vi "Binary Number Mantissa and Exponent (U64).vi"(7 "Binary Number":u64 format="%064b", 9 "Input Valid":bool=TRUE) -> (6 "Exponent (-N)":u8, 8 "Mantissa (M)":u64 format="%.0b", 10 "Output Valid":bool=TRUE)   [LabVIEW 2011]
doc: "This VI computes Mantissa and Exponent of Fixed Point Number\n\n<b> Latency = 8 Ticks </b>"
uses:
  <vilib>/rvi/FXPMathLib/basic elements/FxpDiscreteDelay/XNode/nifxpmath_DiscreteDelay.xnode
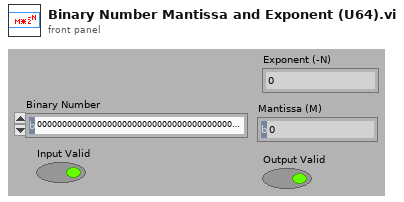
[diagram p1: front panel]
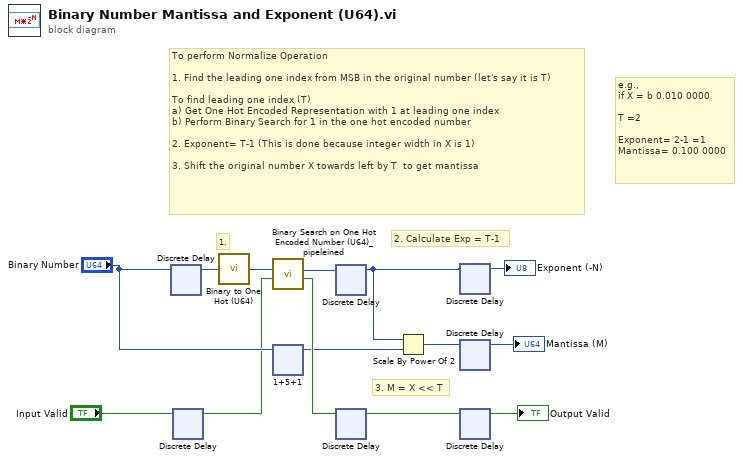
[diagram p0: block diagram]
diagram:
  # "e.g.,\nif X = b 0.010 0000\n\nT =2\n\nExponent= 2-1 =1 \nMantissa= 0.100 0000"
  # "3. M = X << T"
  # "2. Calculate Exp = T-1"
  # "1."
  # "To perform Normalize Operation\n\n1. Find the leading one index from MSB in the original number (let's say it is T)\n\nTo find leading one index (T) \na) Get One Hot Encoded Representation with 1 at leading one index\nb) Perform Binary Search for 1 in the one hot encoded number\n\n2. Exponent= T-1 (This is done because integer width in X is 1)\n\n3. Shift the original number X towards left by T  to get mantissa"
  n1 = xnode "Discrete Delay"("D"="Binary Number") -> ("Q"=w12:u64)
  n2 = xnode "Discrete Delay"("D"="Input Valid") -> ("Q"=w4:bool)
  n3 = call <userlib>:"Binary to One Hot (U64).vi"("Binary Number"=w12) -> ("One Hot Encoded Number"=w5:u64)  [unwired: 14 in]
  n4 = call <userlib>:"Binary Search on One Hot Encoded Number (U64)_pipeleined.vi"("Input Valid"=w4, "One Hot encoded Number"=w5) -> ("Output Valid"=w3:bool, "Binary Number"=w7:u8)  [unwired: 7 in, 1 out]
  n5 = xnode "1+5+1"("D"="Binary Number") -> ("Q"=w2:u64)
  n6 = xnode "Discrete Delay"("D"=w7) -> ("Q"=w1:u8)
  n7 = xnode "Discrete Delay"("D"=w3) -> ("Q"=w10:bool)
  n8 = Scale By Power Of 2(n=w1, x=w2) -> (x*2^n=w6:u64)
  n9 = xnode "Discrete Delay"("D"=w1) -> ("Q"=→"Exponent (-N)":u8)
  n10 = xnode "Discrete Delay"("D"=w6) -> ("Q"=→"Mantissa (M)":u64)
  n11 = xnode "Discrete Delay"("D"=w10) -> ("Q"=→"Output Valid":bool)
